vi "Untitled 122222.vi"() -> ()   [LabVIEW 2010]
uses:
  <vilib>/NXT/Block Support/NXT_InputPort.ctl
  <vilib>/NXT/Subs/MotorOutput.ctl
  <vilib>/NXT/Dual Mode Library/Sensors/Light_On.vi
  <vilib>/NXT/Dual Mode Library/Motors/MotorOn.vi
panel:
  in  "Power (75) 2":i32=75
  in  "stop":bool
  in  "Power (75)":i32=75
  in  "Output Port (All Ports) 2":T1=3 items=["Port A", "Port B", "Port C", "All Ports"]
  in  "Output Port (All Ports)":T1=3 items=["Port A", "Port B", "Port C", "All Ports"]
  in  "Port (Port 3)":T2=2 items=["Port 1", "Port 2", "Port 3", "Port 4"]
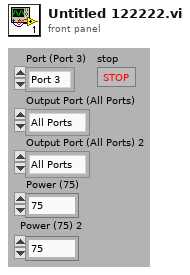
[diagram p1: front panel]
types:
  T1 = typedef "MotorOutput.ctl" = u8
  T2 = typedef "NXT_InputPort.ctl" = u8
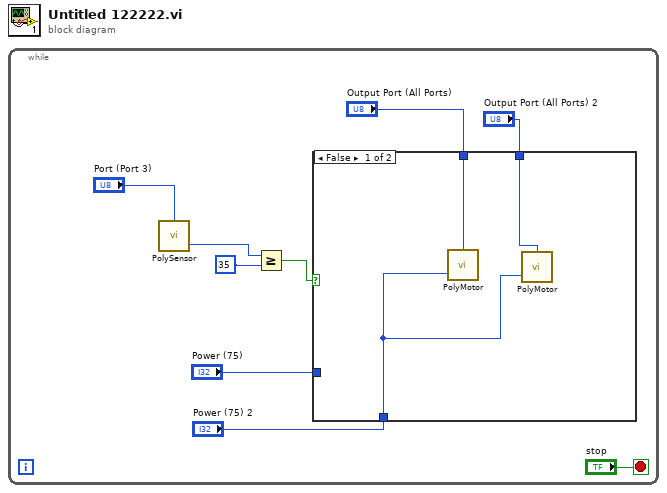
[diagram p0: block diagram]
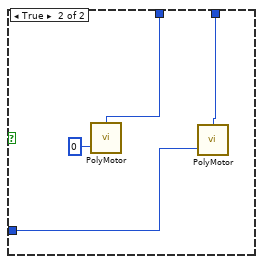
[diagram p2: hidden frame]
diagram:
  n1 = while {
    stop <- "stop" stop-if-true
    n2 = call-poly <vilib>:"PolySensor.vi"("Port (Port 3)"="Port (Port 3)") -> ("Scaled Value"=w5:i16)  [unwired: 2 in, 1 out]
    n3 = Greater Or Equal?(x=w5, y=i16 35 ("Scaled Value")) -> (x >= y?=w9:bool)
    n4 = case shown="False" w9 {
      tunnel: "Output Port (All Ports)" -> [w12 w15]
      tunnel: "Output Port (All Ports) 2" -> [w11 w14]
      tunnel: "Power (75) 2" -> [w10 _]
      tunnel: "Power (75)" -> [_ w13]
      frame False {
        n5 = call-poly <vilib>:"PolyMotor.vi"("Power (75)"=w10, "Output Port (All Ports)"=w12) -> ()  [unwired: 2 in, 1 out]
        n6 = call-poly <vilib>:"PolyMotor.vi"("Power (75)"=w10, "Output Port (All Ports)"=w11) -> ()  [unwired: 2 in, 1 out]
      }
      frame True {
        n7 = call-poly <vilib>:"PolyMotor.vi"("Power (75)"=0, "Output Port (All Ports)"=w15) -> ()  [unwired: 2 in, 1 out]
        n8 = call-poly <vilib>:"PolyMotor.vi"("Power (75)"=w13, "Output Port (All Ports)"=w14) -> ()  [unwired: 2 in, 1 out]
      }
    }
  }
